vi "Make Defect Energy Transition Plot.vi"(6 "Label Spacing":dbl=0.5, 8 "Space Between Lines":dbl=4.5, 9 "Buckets":string[][](array[combo]), 10 "All Defects and Transitions":T1(array[cluster]), 11 "XY Graph Reference":refnum<vi>) -> ()   [LabVIEW 2010]
panel:
  out "Example Graph":cluster{dbl[], dbl[]}[](graph)
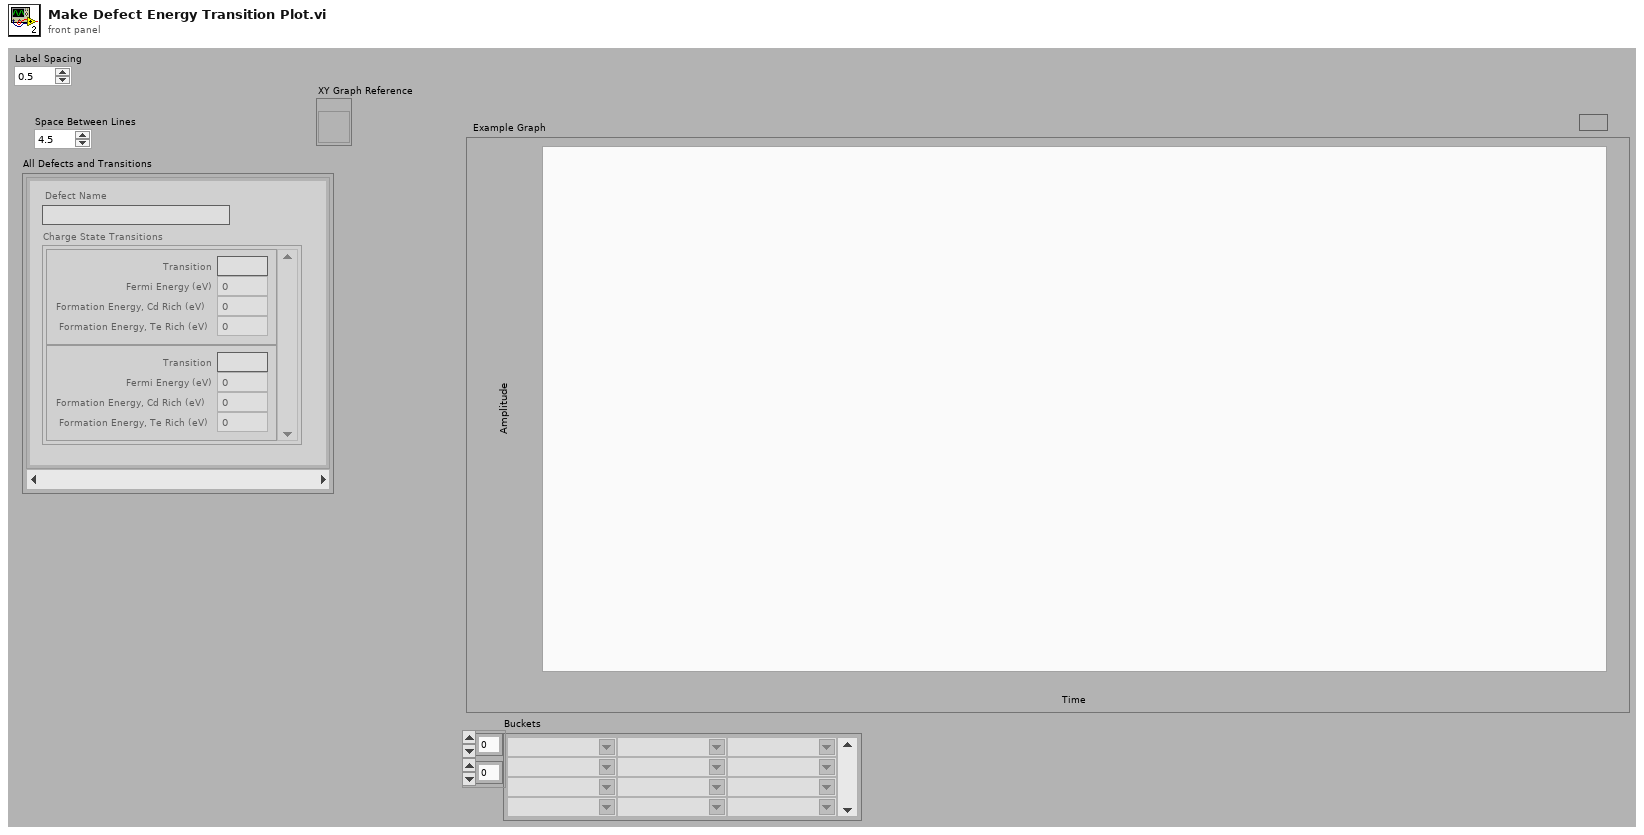
[diagram p1: front panel]
types:
  T1 = cluster{"Defect Name":string, "Charge State Transitions":cluster{"Transition":string, "Fermi Energy (eV)":dbl, "Formation Energy, Cd Rich (eV)":dbl, "Formation Energy, Te Rich (eV)":dbl}[]}[]
  T2 = cluster{"Name":string, "Color":u32, "Style":u8, "Point Style":u8, "Name Visible":bool, "Allow Drag":bool, "Annotation Mode":u32, "Plot":i32, "Index":i32, "Position":cluster{"X":dbl, "Y":dbl}, "X Scale":u32, "Y Scale":u32, "Show Arrow":bool, "Lock Name":bool, "Plot Area":i32, "Label Offset":cluster{"X":dbl, "Y":dbl}}
  T3 = cluster{"Name":string, "Color":u32, "Style":u8, "Point Style":u8, "Name Visible":bool, "Allow Drag":bool, "Annotation Mode":u32, "Plot":i32, "Index":i32, "Position":cluster{"X":dbl, "Y":dbl}, "X Scale":u32, "Y Scale":u32, "Show Arrow":bool, "Lock Name":bool, "Plot Area":i32, "Label Offset":cluster{"X":dbl, "Y":dbl}}[]
  T4 = cluster{"Transition":string, "Fermi Energy (eV)":dbl, "Formation Energy, Cd Rich (eV)":dbl, "Formation Energy, Te Rich (eV)":dbl}[]
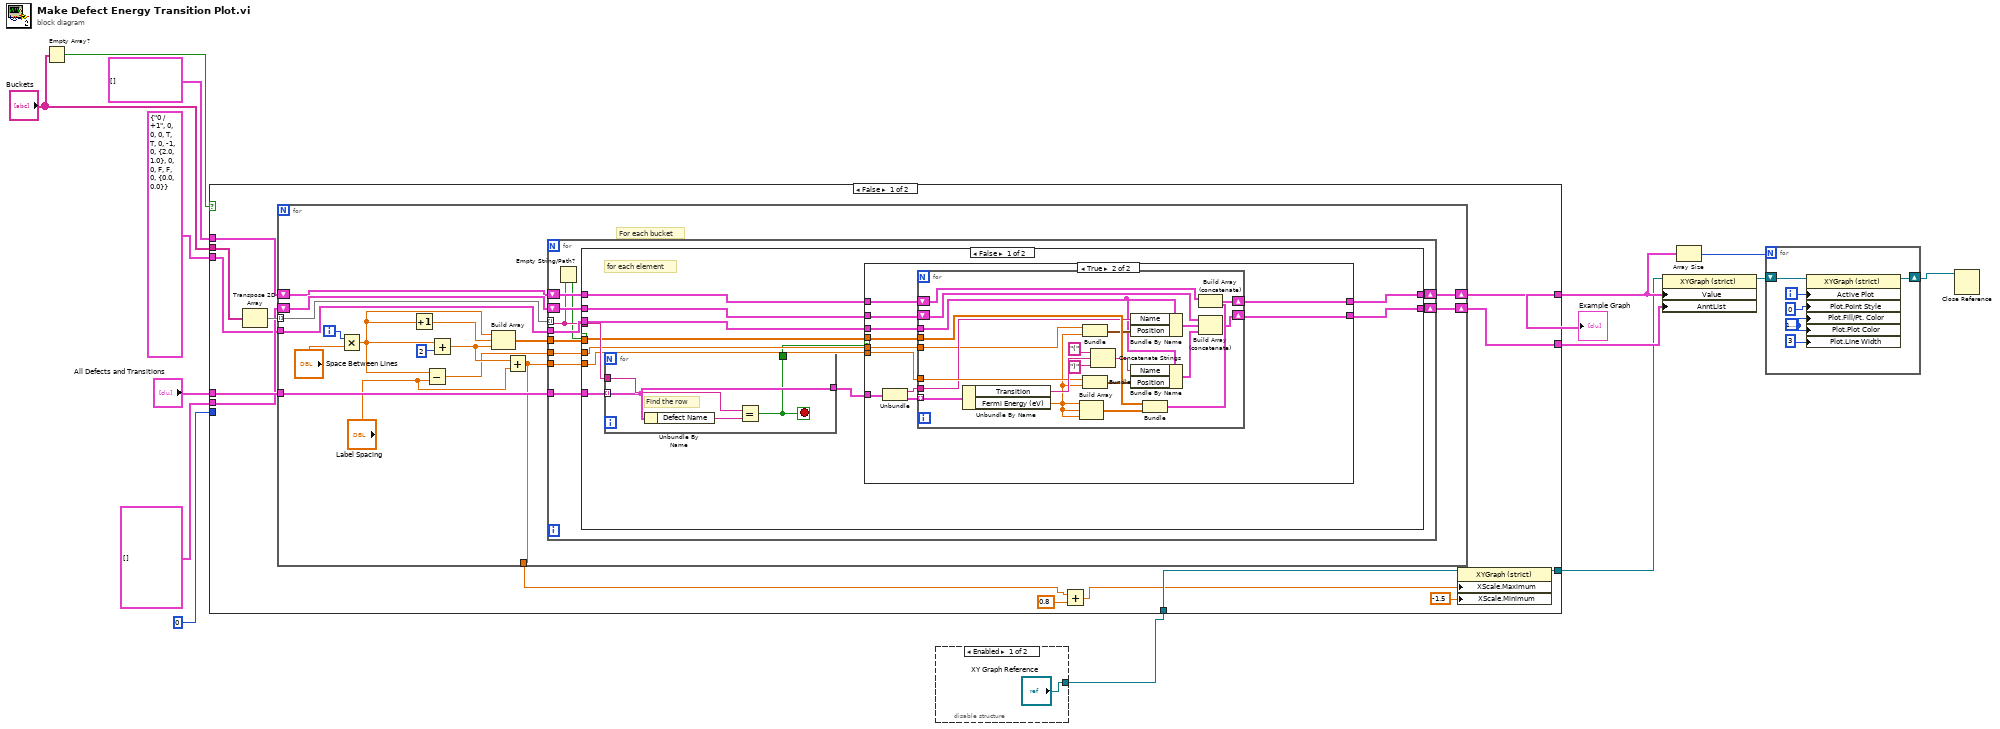
[diagram p0: block diagram]
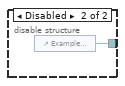
[diagram p2: hidden frame]
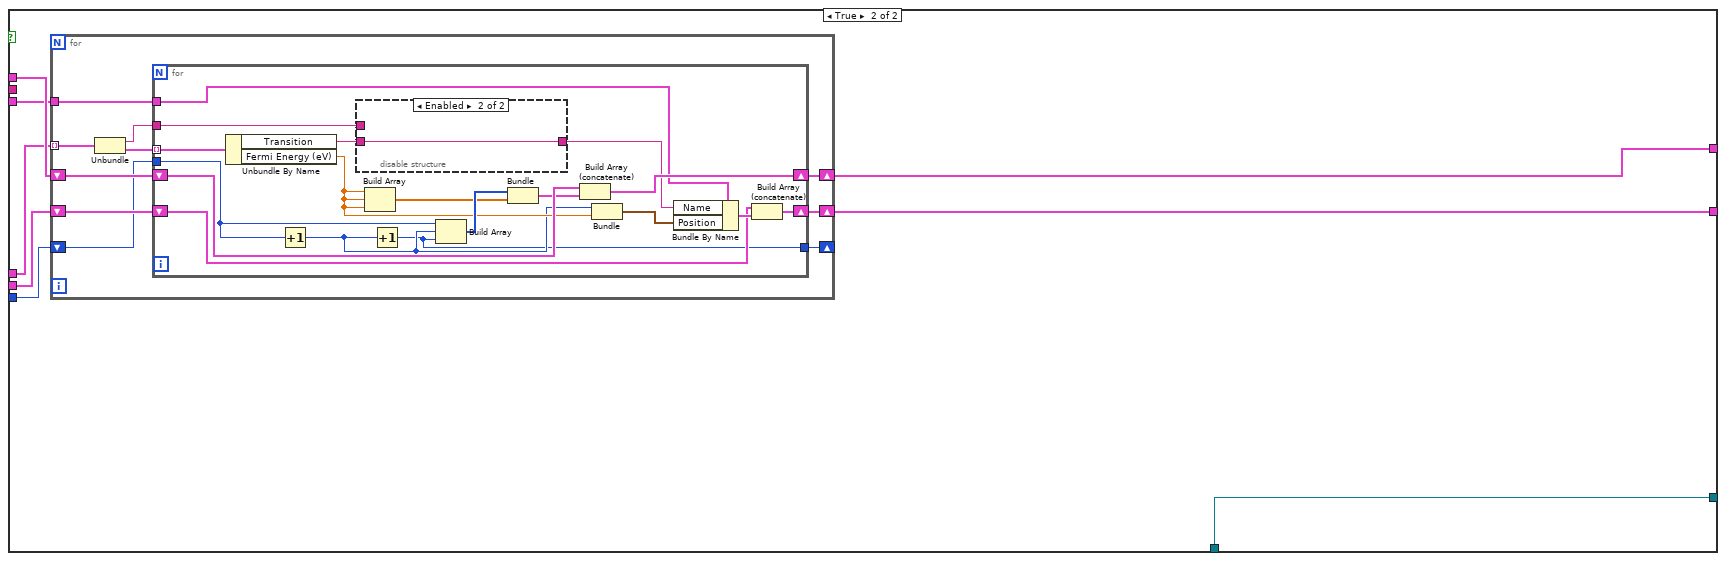
[diagram p5: hidden frame]
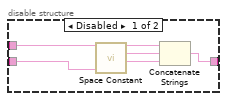
[diagram p6: hidden frame]
diagram:
  n1 = Empty Array?(array="Buckets") -> (empty?=w5:bool)
  n2 = disable-structure shown="Enabled" {
    disable-tunnel: ["XY Graph Reference" w16] -> w3
    frame Enabled {
    }
    frame Disabled {
      n3 = control-ref of="Example Graph"() -> (w16:refnum<vi>)
    }
  }
  n4 = case shown="False" w5 {
    tunnel: cluster{i32[], dbl[]}[] [] -> [w26 w118]
    tunnel: T3 [] -> [w27 w117]
    tunnel: T2 {"Name"="0 / +1", "Color"=0, "Style"=0, "Point Style"=0, "Name Visible"=TRUE, "Allow Drag"=TRUE, "Annotation Mode"=0, "Plot"=-1, "Index"=0, "Position"={"X"=2.0, "Y"=1.0}, "X Scale"=0, "Y Scale"=0, "Show Arrow"=FALSE, "Lock Name"=FALSE, "Plot Area"=0, "Label Offset"={"X"=0.0, "Y"=0.0}} ("element 2") -> [w25 w116]
    tunnel: [w24 w115] -> w11
    tunnel: [w23 w114] -> w10
    tunnel: 0 -> [_ w113]
    tunnel: "All Defects and Transitions" -> [w28 w112]
    tunnel: "Buckets" -> [w30 _]
    tunnel: w3 -> [w22 w111]
    tunnel: [w21 w111] -> w2
    frame False {
      n5 = Transpose 2D Array(2D array=w30) -> (transposed array=w29:string[][])
      n6 = for {
        tunnel: w29 -> [w40] mode=indexing
        tunnel: w28 -> [w47]
        shift-right: [w43] -> w24
        shift-left: w27 -> [w46]
        shift-right: [w44] -> w23
        shift-left: w26 -> [w45]
        tunnel: w25 -> [w42]
        tunnel: [w32] -> w19
        i -> [w41]
        # "For each bucket"
        n7 = Multiply(x=w41, y="Space Between Lines") -> (x*y=w34:dbl)
        n8 = Increment(x=w34) -> (x+1=w39:dbl)
        n9 = Subtract(x=w34, y="Label Spacing") -> (x-y=w33:dbl)
        n10 = Add(x=w34, y=2) -> (x+y=w35:dbl)
        n11 = Build Array(w34, w39, w35) -> (w38:dbl[])
        n12 = Add(x=w35, y="Label Spacing") -> (x+y=w32:dbl)
        n13 = for {
          tunnel: w47 -> [w58]
          tunnel: w40 -> [w49] mode=indexing
          shift-right: [w54] -> w43
          shift-left: w46 -> [w53]
          shift-right: [w56] -> w44
          shift-left: w45 -> [w57]
          tunnel: w42 -> [w55]
          tunnel: w38 -> [w52]
          tunnel: w32 -> [w51]
          tunnel: w33 -> [w50]
          n14 = Empty String/Path?(string/path=w49) -> (empty?=w48:bool)
          n15 = case shown="False" w48 {
            tunnel: w58 -> [w70 _]
            tunnel: w49 -> [w69 _]
            tunnel: w57 -> [w68 w110]
            tunnel: [w67 w110] -> w56
            tunnel: w55 -> [w66 _]
            tunnel: [w64 w109] -> w54
            tunnel: w53 -> [w63 w109]
            tunnel: w52 -> [w62 _]
            tunnel: w51 -> [w61 _]
            tunnel: w50 -> [w60 _]
            frame False {
              # "for each element"
              n16 = for {
                tunnel: w70 -> [w106] mode=indexing
                tunnel: w69 -> [w108]
                tunnel: [w106] -> w65
                tunnel: [w105] -> w59
                stop <- w105 stop-if-true
                # "Find the row"
                n17 = Unbundle By Name(w106) -> ("Defect Name"=w107:string)
                n18 = Equal?(x=w108, y=w107) -> (x = y?=w105:bool)
              }
              n19 = case shown="True" w59 {
                tunnel: w68 -> [w72 w83]
                tunnel: [w72 w82] -> w67
                tunnel: w66 -> [_ w81]
                tunnel: w65 -> [_ w80]
                tunnel: [w71 w78] -> w64
                tunnel: w63 -> [w71 w77]
                tunnel: w62 -> [_ w76]
                tunnel: w61 -> [_ w75]
                tunnel: w60 -> [_ w73]
                frame False {
                }
                frame True {
                  n20 = Unbundle(w80) -> ("Defect Name"=w74:string, "Charge State Transitions"=w79:T4)
                  n21 = for {
                    tunnel: w81 -> [w84]
                    tunnel: w79 -> [w98] mode=indexing
                    shift-right: [w99] -> w82
                    shift-left: w83 -> [w100]
                    shift-right: [w97] -> w78
                    shift-left: w77 -> [w96]
                    tunnel: w76 -> [w95]
                    tunnel: w75 -> [w94]
                    tunnel: w74 -> [w92]
                    tunnel: w73 -> [w88]
                    n22 = Unbundle By Name(w98) -> ("Transition"=w103:string, "Fermi Energy (eV)"=w89:dbl)
                    n23 = Build Array(w89, w89, w89) -> (w104:dbl[])
                    n24 = Bundle(w88, "Fermi Energy (eV)"=w89) -> (w86:cluster{dbl, "Fermi Energy (eV)":dbl})  [unwired: 1 in]
                    n25 = Bundle(w94, "Fermi Energy (eV)"=w89) -> (w87:cluster{dbl, "Fermi Energy (eV)":dbl})  [unwired: 1 in]
                    n26 = Concatenate Strings("(" ("string"), w103, ")" ("string")) -> (w90:string)
                    n27 = Bundle By Name(cluster=w84, "Name"=w92, "Position"=w86) -> (w102:T2)
                    n28 = Bundle By Name(cluster=w84, "Name"=w90, "Position"=w87) -> (w85:T2)
                    n29 = Bundle(w95, w104) -> (w101:cluster{dbl[], dbl[]})  [unwired: 1 in]
                    n30 = Build Array (concatenate)(w100, w101) -> (w99:cluster{dbl[], dbl[]}[])
                    n31 = Build Array (concatenate)(w96, w102, w85) -> (w97:T3)
                  }
                }
              }
            }
            frame True {
            }
          }
        }
      }
      n32 = Add(x=w19, y=0.8) -> (x+y=w17:dbl)
      n33 = property on="Property Node" class="XYGraph (strict)"(reference=w22, "XScale.Maximum"=w17, "XScale.Minimum"=-1.5 ("X Scale.Range:Minimum")) -> (reference out=w21:refnum<vi>)  [unwired: 1 in, 1 out]
    }
    frame True {
      n34 = for {
        tunnel: w112 -> [w128] mode=indexing
        shift-right: [w125] -> w114
        shift-left: w118 -> [w126]
        shift-right: [w121] -> w115
        shift-left: w117 -> [w124]
        tunnel: w116 -> [w123]
        shift-right: [w119] -> _
        shift-left: w113 -> [w120]
        n35 = Unbundle(w128) -> ("Defect Name"=w122:string, "Charge State Transitions"=w127:T4)
        n36 = for {
          tunnel: w127 -> [w146] mode=indexing
          shift-right: [w143] -> w125
          shift-left: w126 -> [w142]
          shift-right: [w137] -> w121
          shift-left: w124 -> [w136]
          tunnel: w123 -> [w141]
          tunnel: w122 -> [w129]
          tunnel: w120 -> [w131]
          tunnel: [w130] -> w119
          n37 = Unbundle By Name(w146) -> ("Transition"=w140:string, "Fermi Energy (eV)"=w133:dbl)
          n38 = Increment(x=w131) -> (x+1=w132:i32)
          n39 = disable-structure shown="Enabled" {
            disable-tunnel: w140 -> [w150 w151]
            disable-tunnel: [w149 w151] -> w139
            disable-tunnel: w129 -> [w147 _]
            frame Disabled {
              n40 = call <vilib>:"Space Constant.vi"() -> ("String"=w148:string)
              n41 = Concatenate Strings(w147, w148, w150) -> (w149:string)
            }
            frame Enabled {
            }
          }
          n42 = Build Array(w133, w133, w133) -> (w144:dbl[])
          n43 = Increment(x=w132) -> (x+1=w130:i32)
          n44 = Build Array(w131, w132, w130) -> (w145:i32[])
          n45 = Bundle(w145, w144) -> (w134:cluster{i32[], dbl[]})  [unwired: 1 in]
          n46 = Build Array (concatenate)(w142, w134) -> (w143:cluster{i32[], dbl[]}[])
          n47 = Bundle(w132, "Fermi Energy (eV)"=w133) -> (w135:cluster{i32, "Fermi Energy (eV)":dbl})  [unwired: 1 in]
          n48 = Bundle By Name(cluster=w141, "Name"=w139, "Position"=w135) -> (w138:T2)
          n49 = Build Array (concatenate)(w136, w138) -> (w137:T3)
        }
      }
    }
  }
  "Example Graph" <- w10
  n50 = property on="Property Node" class="XYGraph (strict)"(reference=w2, "Value"=w10, "AnntList"=w11) -> (reference out=w8:refnum<vi>)  [unwired: 1 in, 1 out]
  n51 = Array Size(array=w10) -> (size(s)=w9:i32)
  n52 = for {
    N: w9 -> [_]
    shift-right: [w152] -> w1
    shift-left: w8 -> [w153]
    i -> [w157]
    w155 = u32 16777222 ("Color Box")
    n53 = property on="Property Node" class="XYGraph (strict)"(reference=w153, "Active Plot"=w157, "Plot.Point Style"=u8 0, "Plot.Fill/Pt. Color"=w155, "Plot.Plot Color"=w155, "Plot.Line Width"=u8 3) -> (reference out=w152:refnum<vi>)  [unwired: 1 in, 1 out]
  }
  n54 = Close Reference(reference=w1) -> ()  [unwired: 1 in, 1 out]
